vi "Auton-ZeroEverything.vi"(8 "error in (no error)":errorcluster, 11 "Auton Event Queue Data":refnum<queue>) -> (0 "error out":errorcluster, 2 "Done?":bool, 3 "Auton Event Queue Data 2":refnum<queue>)   [LabVIEW 2014]
uses:
  Robot Global Data.vi
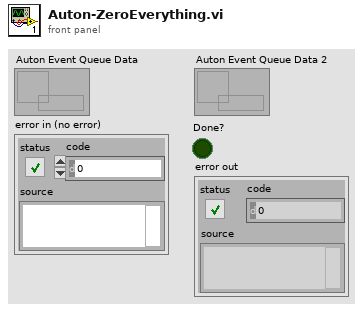
[diagram p1: front panel]
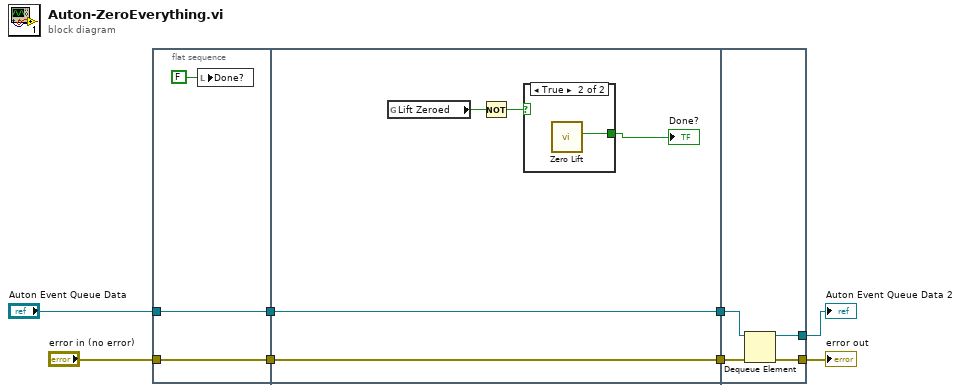
[diagram p0: block diagram]
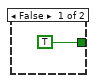
[diagram p2: hidden frame]
diagram:
  n1 = flat-sequence {
    tunnel: [w10] -> w8
    tunnel: "error in (no error)" -> [w10]
    tunnel: [w9] -> w6
    tunnel: "Auton Event Queue Data" -> [w9]
    tunnel: w8 -> [w13]
    tunnel: w6 -> [w14]
    tunnel: [w14] -> w4
    tunnel: [w13] -> w2
    tunnel: w4 -> [w22]
    tunnel: [w21] -> w3
    tunnel: w2 -> [w20]
    tunnel: [w19] -> w1
    frame #0 {
      n2 = local write "Done?"(FALSE ("Done?")) -> ()
    }
    frame #1 {
      n3 = global read "Robot Global Data.vi" "Lift Zeroed"() -> (w16:bool)
      n4 = Not(x=w16) -> (.not. x?=w15:bool)
      n5 = case shown="True" w15 {
        tunnel: [TRUE w18] -> w12
        frame False {
        }
        frame True {
          n6 = call "Zero Lift.vi"() -> ("Boolean"=w18:bool)  [unwired: 11 in]
        }
      }
      "Done?" <- w12
    }
    frame #2 {
      n7 = Dequeue Element(queue=w22, error in (no error)=w20) -> (queue out=w21:refnum<queue>, error out=w19:errorcluster)  [unwired: 1 in, 2 out]
    }
  }
  "Auton Event Queue Data 2" <- w3
  "error out" <- w1
